vi "Set_shutdown_HV.vi"() -> ()   [LabVIEW 2012]
uses:
  hv cluster control.ctl
  <vilib>/Platform/TimedLoop/XDataNode/timing_clust.ctl
  <vilib>/Platform/TimedLoop/XDataNode/nitl_modes.ctl
  <vilib>/Platform/TimedLoop/XDataNode/wakeup.ctl
  <vilib>/Platform/TimedLoop/XDataNode/XDataNode.xnode
  Program Files/CAEN/HV/CAENHVWrapper/labview/CAENHVWrapper/CAENHVWrapper.lvlib
  <vilib>/Platform/TimedLoop/XDataNode/XDNodeRunTimeDep.lvlib
panel:
  out "Current(uA)":sgl[](array[numeric])
  out "HV (V)":sgl[](array[numeric])
  in  "stop":bool
  in  "Set the HVs":bool=TRUE
  in  "HV Power On/Off":bool[](array[boolean])=[TRUE, TRUE, TRUE, TRUE, TRUE, TRUE, TRUE, TRUE]
  in  "HV Tolerance (%)":dbl=1.0
  in  "Set Voltage":string[](array[string])=["718", "586", "680", "700", "990", "670", "690", "760"]
  out "handle":i32
  in  "IP adress HV2":string="1_0_0"
  in  "IP adress HV1":string="0_0_0"
  in  "HV Cluster":T1={"HV Power On/Off"=[TRUE, TRUE], "Set Voltage"=["0", "0", "0", "0", "0", "0", "0", "0"], "HV Tolerance (%)"=1.0}
  # "Turn off HVs"
  # "This VI is needed to set the\nvoltages of the HV and turning channels on or off. The settings are directly fed with 'shared variables'\nto the Host program."
  # "Channel 0"
  # "The IP adress of the High Voltages depends on how you connected the two CAEN HVs, you can test which one  is which by first turning on the first 4 \nchannels and see which HV is turned on, this should then be HV1.\n\nWhen you want to shut down the HVs, just turn the switch to 'Turn off HVs' and run the VI."
  # "Channel 1"
  # "Channel 2"
  # "Channel 3"
  # "Channel 4"
  # "Channel 5"
  # "Channel 6"
  # "Channel 7"
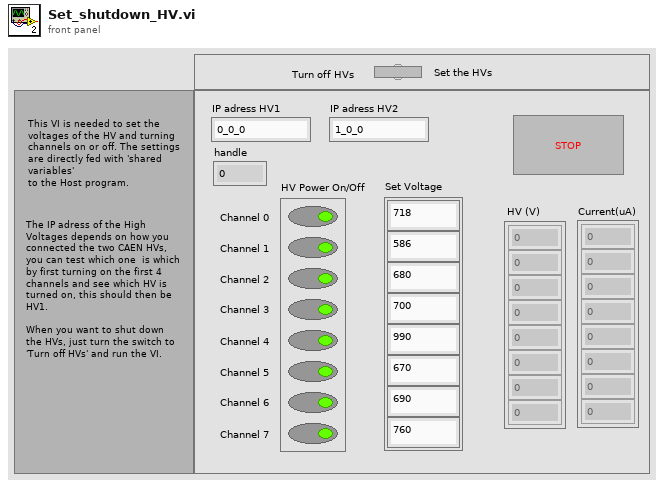
[diagram p1: front panel]
types:
  T1 = typedef "hv cluster control.ctl" = cluster{"HV Power On/Off":bool[], "Set Voltage":string[], "HV Tolerance (%)":dbl}
  T2 = typedef "XDNodeRunTimeDep.lvlib/timing_clust.ctl" = cluster{"Expected End [f-1]":u64, "Actual End [f-1]":u64, "Finished Late? [f-1]":bool, "Expected End [i-1]":u64, "Actual End [i-1]":u64, "Finished Late? [i-1]":bool, "Expected Start [i]":u64, "Actual Start [i]":u64, "Expected Start [f]":u64, "Actual Start [f]":u64, "Source Name":string, "Structure Name":string, "Period":i64, "Deadline":i64, "Offset":i64, "Start":i64, "Priority":i32, "Timeout":i32, "Mode":T3, "Wakeup Reason":T4, "Error":errorcluster, "Source Type":string, "Secondary Source Type":string, "Global End Time":u64, "Global Start Time":u64, "Frame Duration":u64, "Iteration Duration":u64, "Assigned CPU":i32, "I/O Scan Engine Mode":u32}
  T3 = typedef "XDNodeRunTimeDep.lvlib/nitl_modes.ctl" = enum32{"No Change", "Process missed periods, maintain original phase", "Discard missed periods, maintain original phase", "Process missed periods, ignore original phase", "Discard missed periods, ignore original phase"}
  T4 = typedef "XDNodeRunTimeDep.lvlib/wakeup.ctl" = enum32{"Normal", "Aborted", "Asynchronous wakeup", "Timing source error", "Timed loop error", "Timeout"}
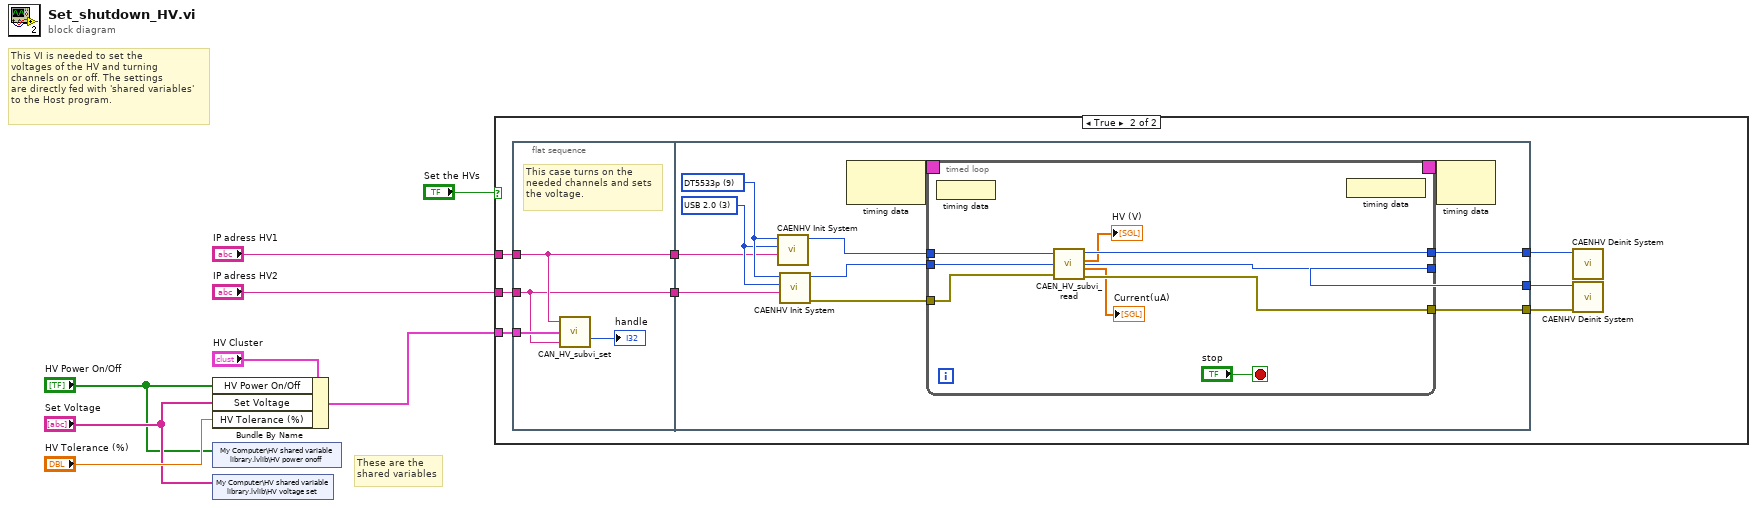
[diagram p0: block diagram]
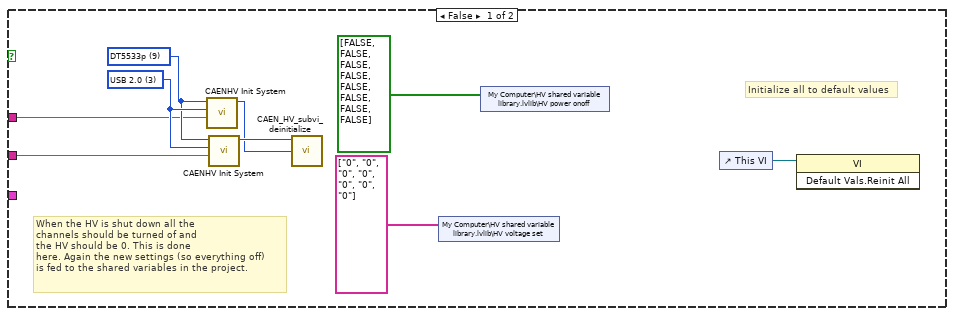
[diagram p2: hidden frame]
diagram:
  # "These are the\nshared variables"
  # "This VI is needed to set the\nvoltages of the HV and turning \nchannels on or off. The settings \nare directly fed with 'shared variables'\nto the Host program."
  n1 = Bundle By Name(cluster="HV Cluster", "HV Power On/Off"="HV Power On/Off", "Set Voltage"="Set Voltage", "HV Tolerance (%)"="HV Tolerance (%)") -> (w6:T1)
  n2 = shared-variable "My Computer\\HV shared variable library.lvlib\\HV power onoff"("HV Power On/Off") -> ()  [unwired: 1 in, 1 out]
  n3 = shared-variable "My Computer\\HV shared variable library.lvlib\\HV voltage set"("Set Voltage") -> ()  [unwired: 1 in, 1 out]
  n4 = case shown="True" "Set the HVs" {
    tunnel: "IP adress HV1" -> [w13 w24]
    tunnel: "IP adress HV2" -> [w12 w23]
    tunnel: w6 -> [_ w25]
    frame False {
      w17 = 3 items=["TCP/IP"=0, "HS CAENET"=2, "USB 2.0"=3, "CONET Optical Link"=4, "USB VCP"=5] ("LinkType")
      w16 = u32 9 items=["SY1527", "SY2527", "SY4527", "SY5527", "N568", "V65XX", "N1470", "V8100", "", "DT5533p"] ("system")
      # "When the HV is shut down all the\nchannels should be turned of and \nthe HV should be 0. This is done \nhere. Again the new settings (so everything off)\nis fed to the shared variables in the project."
      # "Initialize all to default values"
      n5 = call "CAENHV Init System.vi"("Arg"=w13, "LinkType"=w17, "system"=w16) -> ("handle"=w14:i32)  [unwired: 7 in, 1 out]
      n6 = call "CAENHV Init System.vi"("Arg"=w12, "LinkType"=w17, "system"=w16) -> ("handle"=w15:i32)  [unwired: 7 in, 1 out]
      n7 = call "CAEN_HV_subvi_deinitialize.vi"("Handle 2"=w15, "Handle 1"=w14) -> ()  [unwired: 1 in, 1 out]
      n8 = shared-variable "My Computer\\HV shared variable library.lvlib\\HV voltage set"(string[] ["0", "0", "0", "0", "0", "0", "0"]) -> ()  [unwired: 1 in, 1 out]
      n9 = shared-variable "My Computer\\HV shared variable library.lvlib\\HV power onoff"(bool[] [FALSE, FALSE, FALSE, FALSE, FALSE, FALSE, FALSE, FALSE]) -> ()  [unwired: 1 in, 1 out]
      n10 = control-ref of="This VI"() -> (w11:refnum<vi>)
      n11 = invoke class="VI" method="Default Vals.Reinit All"(reference=w11) -> ()  [unwired: 2 in, 3 out]
    }
    frame True {
      n12 = flat-sequence {
        tunnel: w25 -> [w28]
        tunnel: w24 -> [w27]
        tunnel: w23 -> [w26]
        tunnel: [w27] -> w22
        tunnel: [w26] -> w21
        tunnel: w22 -> [w35]
        tunnel: w21 -> [w34]
        tunnel: [w32] -> w20
        tunnel: [w31] -> w19
        tunnel: [w30] -> w18
        frame #0 {
          # "This case turns on the\nneeded channels and sets\nthe voltage."
          n13 = call "CAN_HV_subvi_set.vi"("IP adress HV2"=w26, "HV Cluster"=w28, "IP adress HV1"=w27) -> ("handle"=→"handle":i32)  [unwired: 1 out]
        }
        frame #1 {
          w36 = 3 items=["TCP/IP"=0, "HS CAENET"=2, "USB 2.0"=3, "CONET Optical Link"=4, "USB VCP"=5] ("LinkType")
          w37 = u32 9 items=["SY1527", "SY2527", "SY4527", "SY5527", "N568", "V65XX", "N1470", "V8100", "", "DT5533p"] ("system")
          n14 = call "CAENHV Init System.vi"("Arg"=w35, "LinkType"=w36, "system"=w37) -> ("handle"=w38:i32)  [unwired: 7 in, 1 out]
          n15 = call "CAENHV Init System.vi"("Arg"=w34, "LinkType"=w36, "system"=w37) -> ("error out"=w33:errorcluster, "handle"=w39:i32)  [unwired: 7 in]
          n16 = node-c288() -> (w41:T2)  [unwired: 1 in]
          n17 = timed-loop {
            timing: w41 -> [_]
            timing-out: [_] -> w40
            tunnel: w38 -> [w49]
            tunnel: w39 -> [w48]
            tunnel: w33 -> [w47]
            tunnel: [w46] -> w32
            tunnel: [w45] -> w31
            tunnel: [w44] -> w30
            stop <- "stop" stop-if-true
            n18 = node-c288() -> ()  [unwired: 1 in]
            n19 = call "CAEN_HV_subvi_read.vi"("handle HV1"=w49, "handle HV2"=w48, "error in (no error)"=w47) -> ("handle HV1 out"=w46:i32, "HV"=→"HV (V)":sgl[], "Current"=→"Current(uA)":sgl[], "error out"=w44:errorcluster, "handle HV2 out"=w45:i32)
            n20 = node-c288() -> ()  [unwired: 1 out]
          }
          n21 = node-c288(w40) -> ()  [unwired: 1 out]
        }
      }
      n22 = call "CAENHV Deinit System.vi"("handle"=w20) -> ()  [unwired: 10 in, 1 out]
      n23 = call "CAENHV Deinit System.vi"("error in (no error)"=w18, "handle"=w19) -> ()  [unwired: 9 in, 1 out]
    }
  }
